vi "Get Neurons Info.vi"(10 "Neuron No":i32, 11 "Grid in":refnum<class "Grid.lvclass">) -> (0 "Active":bool, 1 "Position":i32[](array[numeric]), 2 "Group":T1, 3 "Grid out":refnum<class "Grid.lvclass">, 4 "Neuron Id":i32, 5 "Size radio (um)":dbl, 6 "Color":u32(colorbox))   [LabVIEW 2016, in "Grid.lvclass"]
doc: "Get the information of an specific neuron in the grid"
uses:
  Grid.lvclass
  Controls/Type of Neuron.ctl
  Grid.lvclass/Grid.ctl
  Neuron/Neuron.lvclass/Neuron.ctl
  Neuron/Neuron.lvclass
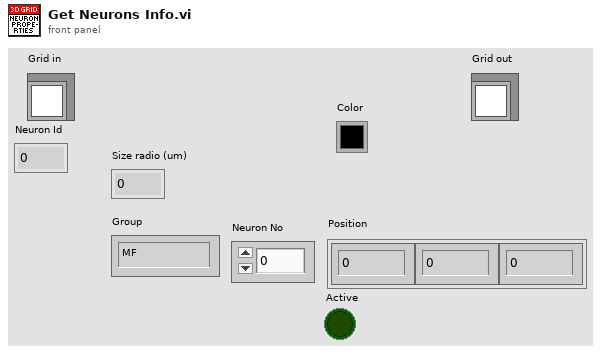
[diagram p1: front panel]
types:
  T1 = typedef "Type of Neuron.ctl" = enum16{"MF", "BA", "GO", "GC", "PC", "LU", "Glia (Dummy)"}
  T2 = typedef "Neuron Info.ctl" = cluster{"N":i32, "Radius":dbl, "Type":T1, "Color":u32}[]
  T3 = cluster{"N":i32, "Radius":dbl, "Type":T1, "Color":u32}
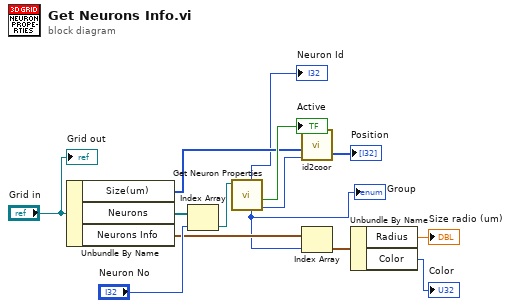
[diagram p0: block diagram]
diagram:
  n1 = Unbundle By Name("Grid in") -> ("Size(um)"=w5:u32[], "Neurons"=w11:refnum<class "Neuron.lvclass">[], "Neurons Info"=w9:T2)
  n2 = Index Array(array=w11, index="Neuron No") -> (element=w12:refnum<class "Neuron.lvclass">)
  n3 = call "Get Neuron Properties.vi"("Neuron in"=w12) -> ("Position Key"=w4:i32, "Active"=→"Active":bool, "Group"=w6:T1, "ID"=→"Neuron Id":i32)  [unwired: 5 in, 2 out]
  "Group" <- w6
  n4 = call "id2coor.vi"("Id"=w4, "Size (x,y,z)"=w5) -> ("Position (x,y,z)"=→"Position":i32[])  [unwired: 3 in]
  n5 = Index Array(array=w9, index=w6) -> (element=w8:T3)
  n6 = Unbundle By Name(w8) -> ("Radius"=→"Size radio (um)":dbl, "Color"=→"Color":u32)
  "Grid out" <- "Grid in"
